vi "Export - Tx Packet.vi"(8 "error in (no error)":errorcluster, 11 "Device Item Ref in":T13 format="%.0x") -> (0 "error out":errorcluster, 3 "Tx Packet":T1 {"threadOptions"."pclDecimation" max=16 step=1; "threadOptions"."loopPeriod" max=16 step=1; "threadOptions"."targetPriority" min=-2 max=16 step=1; "threadOptions"."targetProcessor" min=-2 max=16 step=1; "Endianness" items=["big-endian"=0, "little-endian"=2]})   [LabVIEW 2019, in "UDP-Custom-Device System Explorer.lvlib"]
uses:
  UDP-Custom-Device System Explorer.lvlib
  <vilib>/NI VeriStand/Custom Device API/Custom Device Item Ref.ctl
  Types/XML - New/ImpExp - Tx Packet Data.ctl
  <vilib>/NI VeriStand/Custom Device API/Custom Device Item Info.ctl
  Shared/Types/Shared - Channel Data Type.ctl
  Shared/Types/Shared - Buffered.PacketInfo.ctl
  Shared/Types/Shared - Pointer Encoding.ctl
  Shared/Types/Shared - Receive Buffer Options.ctl
  Shared/Types/Shared - Transmit Buffer Options.ctl
  Shared/Types/Shared - Transmit Flag Options.ctl
  Shared/Types/Shared - Transmit Echo Options.ctl
  Types/Threading/Thread Configuration.ctl
  Types/Threading/Thread Sync Reference.ctl
  Shared/Types/Shared - Thread Management.ctl
  Property Accessors/Shared Packet Accessors.lvlib
  Property Accessors/Tx Packet Accessors.lvlib
  <vilib>/NI VeriStand/Custom Device API/Custom Device API.lvlib
  Shared/UDP-Custom-Device Shared.lvlib
  <vilib>/NI VeriStand/Custom Device Tools/Custom Device Utility Library/Custom Device Utility Library.lvlib
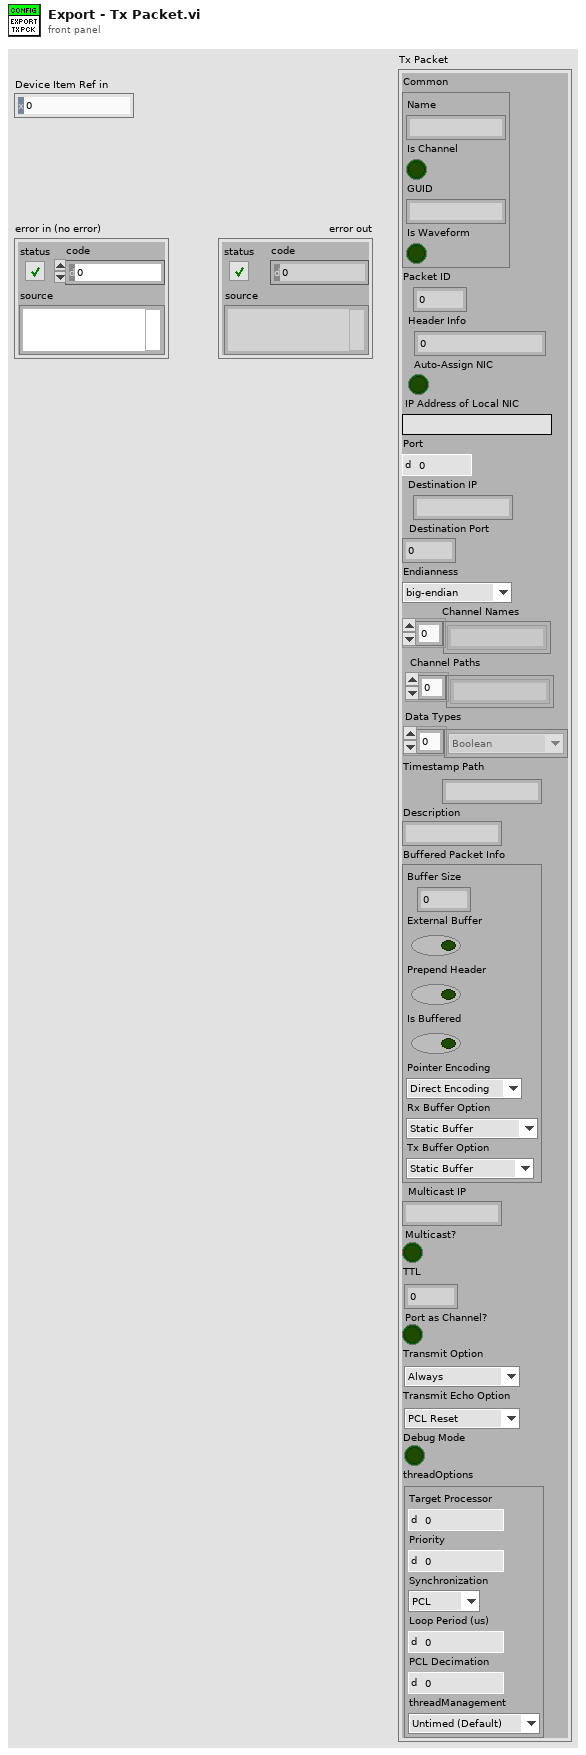
[diagram p1: front panel]
types:
  T1 = typedef "UDP-Custom-Device System Explorer.lvlib/ImpExp - Tx Packet Data.ctl" = cluster{"Common":T2, "Packet ID":i32, "Header Info":u32, "Auto-Assign NIC":bool, "IP Address of Local NIC":string, "Port":u16, "Destination IP":string, "Destination Port":u16, "Endianness":u16, "Channel Names":string[], "Channel Paths":string[], "Data Types":T3[], "Timestamp Path":string, "Description":string, "Buffered Packet Info":T4, "Multicast IP":string, "Multicast?":bool, "TTL":u16, "Port as Channel?":bool, "Transmit Option":T8, "Transmit Echo Option":T9, "Debug Mode":bool, "threadOptions":T10}
  T2 = typedef "Custom Device API.lvlib/Custom Device Item Info.ctl" = cluster{"Name":string, "Is Channel":bool, "GUID":string, "Is Waveform":bool}
  T3 = typedef "UDP-Custom-Device Shared.lvlib/Shared - Channel Data Type.ctl" = enum16{"Boolean", "Single", "Double", "I8", "I16", "I32", "I64", "U8", "U16", "U32", "U64"}
  T4 = typedef "UDP-Custom-Device Shared.lvlib/Shared - Buffered.PacketInfo.ctl" = cluster{"Buffer Size":i32, "External Buffer":bool, "Prepend Header":bool, "Is Buffered":bool, "Pointer Encoding":T5, "Rx Buffer Option":T6, "Tx Buffer Option":T7}
  T5 = typedef "UDP-Custom-Device Shared.lvlib/Shared - Pointer Encoding.ctl" = enum16{"Direct Encoding", "Conversion Encoding"}
  T6 = typedef "UDP-Custom-Device Shared.lvlib/Shared - Receive Buffer Options.ctl" = enum16{"Static Buffer", "Circular Buffer", "Circular Buffer + Size", "Internal Cache", "Internal Cache + Size", "Ping Pong", "Ping Pong + Size"}
  T7 = typedef "UDP-Custom-Device Shared.lvlib/Shared - Transmit Buffer Options.ctl" = enum16{"Static Buffer", "FIFO Buffer", "FIFO Buffer + Port"}
  T8 = typedef "UDP-Custom-Device Shared.lvlib/Shared - Transmit Flag Options.ctl" = enum16{"Always", "One-Shot", "Toggle"}
  T9 = typedef "UDP-Custom-Device Shared.lvlib/Shared - Transmit Echo Options.ctl" = enum16{"PCL Reset", "Counter", "Mirror"}
  T10 = typedef "UDP-Custom-Device System Explorer.lvlib/Thread Configuration.ctl" = cluster{"targetProcessor":i8, "targetPriority":i16, "Synchronization":T11, "loopPeriod":u32, "pclDecimation":u16, "threadManagement":T12}
  T11 = typedef "UDP-Custom-Device System Explorer.lvlib/Thread Sync Reference.ctl" = enum16{"PCL", "Async"}
  T12 = typedef "UDP-Custom-Device Shared.lvlib/Shared - Thread Management.ctl" = enum16{"Untimed (Default)", "Timed (High Priority)"}
  T13 = typedef "Custom Device API.lvlib/Custom Device Item Ref.ctl" = u64
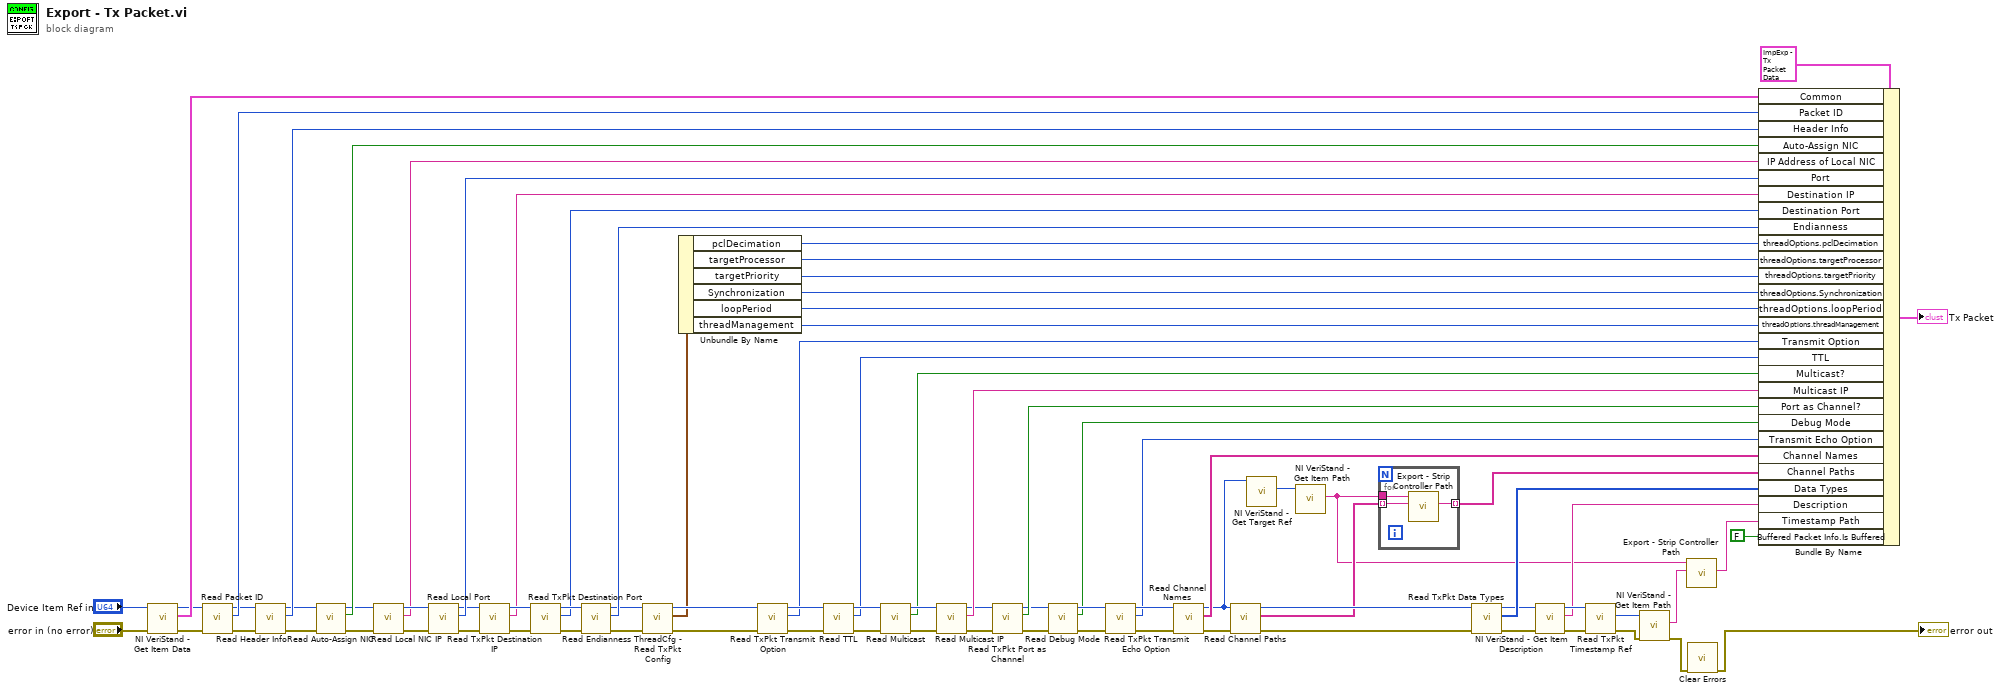
[diagram p0: block diagram]
diagram:
  n1 = call <vilib>:"NI VeriStand - Get Item Data.vi"("error in (no error)"="error in (no error)", "Item Ref in"="Device Item Ref in") -> ("error out"=w49:errorcluster, "Item Info"=w80:T2, "Item Ref out"=w79:T13)  [unwired: 6 in, 1 out]
  n2 = call "Read Packet ID.vi"("error in (no error)"=w49, "Node Ptr"=w79) -> ("error out"=w76:errorcluster, "Packet ID"=w78:i32, "Node Ptr out"=w77:T13)  [unwired: 7 in]
  n3 = call "Read Header Info.vi"("error in (no error)"=w76, "Node Ptr"=w77) -> ("error out"=w73:errorcluster, "Header Info"=w75:u32, "Node Ptr out"=w74:T13)  [unwired: 7 in]
  n4 = call "Read Auto-Assign NIC.vi"("error in (no error)"=w73, "Node Ptr"=w74) -> ("error out"=w68:errorcluster, "Auto-Assign NIC"=w72:bool, "Node Ptr out"=w71:T13)  [unwired: 7 in]
  n5 = call "Read Local NIC IP.vi"("error in (no error)"=w68, "Node Ptr"=w71) -> ("error out"=w69:errorcluster, "IP Address of Local NIC"=w67:string, "Node Ptr out"=w70:T13)  [unwired: 7 in]
  n6 = call "Read Local Port.vi"("error in (no error)"=w69, "Node Ptr"=w70) -> ("error out"=w64:errorcluster, "Port"=w66:u16, "Node Ptr out"=w65:T13)  [unwired: 7 in]
  n7 = call "Read TxPkt Destination IP.vi"("error in (no error)"=w64, "Node Ptr"=w65) -> ("error out"=w62:errorcluster, "Destination IP"=w59:string, "Node Ptr out"=w63:T13)  [unwired: 7 in]
  n8 = call "Read TxPkt Destination Port.vi"("error in (no error)"=w62, "Node Ptr"=w63) -> ("error out"=w60:errorcluster, "Destination Port"=w58:u16, "Node Ptr out"=w61:T13)  [unwired: 7 in]
  n9 = call "Read Endianness.vi"("error in (no error)"=w60, "Node Ptr"=w61) -> ("error out"=w8:errorcluster, "Endianness"=w57:u16, "Node Ptr out"=w9:T13)  [unwired: 7 in]
  n10 = call "ThreadCfg - Read TxPkt Config.vi"("error in (no error)"=w8, "Node Ptr In"=w9) -> ("error out"=w11:errorcluster, "threadOptions"=w7:T10, "Node Ptr Out"=w10:T13)  [unwired: 7 in]
  n11 = Unbundle By Name(w7) -> ("pclDecimation"=w6:u16, "targetProcessor"=w5:i8, "targetPriority"=w4:i16, "Synchronization"=w3:T11, "loopPeriod"=w2:u32, "threadManagement"=w1:T12)
  n12 = call "Read TxPkt Transmit Option.vi"("error in (no error)"=w11, "Node Ptr"=w10) -> ("error out"=w21:errorcluster, "Transmit Options"=w20:T8, "Node Ptr out"=w22:T13)  [unwired: 7 in]
  n13 = call "Read TTL.vi"("error in (no error)"=w21, "Node Ptr"=w22) -> ("error out"=w33:errorcluster, "TTL"=w29:u16, "Node Ptr out"=w32:T13)  [unwired: 7 in]
  n14 = call "Read Multicast.vi"("error in (no error)"=w33, "Node Ptr"=w32) -> ("error out"=w30:errorcluster, "Multicast"=w28:bool, "Node Ptr out"=w31:T13)  [unwired: 7 in]
  n15 = call "Read Multicast IP.vi"("error in (no error)"=w30, "Node Ptr"=w31) -> ("error out"=w24:errorcluster, "Multicast IP Address"=w27:string, "Node Ptr out"=w25:T13)  [unwired: 7 in]
  n16 = call "Read TxPkt Port as Channel.vi"("error in (no error)"=w24, "Node Ptr"=w25) -> ("error out"=w14:errorcluster, "Port as Channel"=w23:bool, "Node Ptr out"=w16:T13)  [unwired: 7 in]
  n17 = call "Read Debug Mode.vi"("error in (no error)"=w14, "Node Ptr"=w16) -> ("error out"=w13:errorcluster, "Debug Mode"=w12:bool, "Node Ptr out"=w15:T13)  [unwired: 7 in]
  n18 = call "Read TxPkt Transmit Echo Option.vi"("error in (no error)"=w13, "Node Ptr"=w15) -> ("error out"=w19:errorcluster, "Transmit Echo Options"=w17:T9, "Node Ptr out"=w18:T13)  [unwired: 7 in]
  n19 = call "Read Channel Names.vi"("error in (no error)"=w19, "Node Ptr"=w18) -> ("error out"=w56:errorcluster, "Channel Names"=w55:string[], "Node Ptr out"=w39:T13)  [unwired: 7 in]
  n20 = call "Read Channel Paths.vi"("error in (no error)"=w56, "Node Ptr"=w39) -> ("error out"=w53:errorcluster, "Channel Paths"=w38:string[], "Node Ptr out"=w54:T13)  [unwired: 7 in]
  n21 = call <vilib>:"NI VeriStand - Get Target Ref.vi"("Item Ref in"=w39) -> ("Target Ref"=w40:T13)  [unwired: 7 in, 3 out]
  n22 = call <vilib>:"NI VeriStand - Get Item Path.vi"("Item Ref in"=w40) -> ("Path"=w36:string)  [unwired: 7 in, 3 out]
  n23 = for {
    tunnel: w38 -> [w86] mode=indexing
    tunnel: w36 -> [w85]
    tunnel: [w84] -> w37 mode=indexing
    n24 = call "Export - Strip Controller Path.vi"("Channel Path"=w86, "Controller Path"=w85) -> ("Stripped Path"=w84:string)  [unwired: 8 in, 1 out]
  }
  n25 = call "Read TxPkt Data Types.vi"("error in (no error)"=w53, "Node Ptr"=w54) -> ("error out"=w43:errorcluster, "Data types"=w52:T3[], "Node Ptr out"=w45:T13)  [unwired: 7 in]
  n26 = call <vilib>:"NI VeriStand - Get Item Description.vi"("error in (no error)"=w43, "Item Ref in"=w45) -> ("error out"=w42:errorcluster, "Description"=w41:string, "Item Ref out"=w44:T13)  [unwired: 6 in, 1 out]
  n27 = call "Read TxPkt Timestamp Ref.vi"("error in (no error)"=w42, "Node Ptr"=w44) -> ("error out"=w50:errorcluster, "Timestamp Ref"=w51:T13)  [unwired: 7 in, 1 out]
  n28 = call <vilib>:"NI VeriStand - Get Item Path.vi"("error in (no error)"=w50, "Item Ref in"=w51) -> ("error out"=w48:errorcluster, "Path"=w35:string)  [unwired: 6 in, 2 out]
  n29 = call "Export - Strip Controller Path.vi"("Channel Path"=w35, "Controller Path"=w36) -> ("Stripped Path"=w34:string)  [unwired: 8 in, 1 out]
  n30 = call <vilib>:"Clear Errors.vi"("error in (no error)"=w48) -> ("error out"=→"error out":errorcluster)  [unwired: 5 in, 1 out]
  n31 = Bundle By Name(cluster=T1 {"Common"={"Name"="", "Is Channel"=FALSE, "GUID"="", "Is Waveform"=FALSE}, "Packet ID"=0, "Header Info"=0, "Auto-Assign NIC"=FALSE, "IP Address of Local NIC"="", "Port"=0, "Destination IP"="", "Destination Port"=0, "Endianness"=0, "Channel Names"=[], "Channel Paths"=[], "Data Types"=[], "Timestamp Path"="", "Description"="", "Buffered Packet Info"={"Buffer Size"=0, "External Buffer"=FALSE, "Prepend Header"=FALSE, "Is Buffered"=FALSE, "Pointer Encoding"=enum."Direct Encoding", "Rx Buffer Option"=enum."Static Buffer", "Tx Buffer Option"=enum."Static Buffer"}, "Multicast IP"="", "Multicast?"=FALSE, "TTL"=0, "Port as Channel?"=FALSE, "Transmit Option"=enum."Always", "Transmit Echo Option"=enum."PCL Reset", "Debug Mode"=FALSE, "threadOptions"={"targetProcessor"=0, "targetPriority"=0, "Synchronization"=enum."PCL", "loopPeriod"=0, "pclDecimation"=0, "threadManagement"=enum."Untimed (Default)"}} ("Tx Packet"), "Common"=w80, "Packet ID"=w78, "Header Info"=w75, "Auto-Assign NIC"=w72, "IP Address of Local NIC"=w67, "Port"=w66, "Destination IP"=w59, "Destination Port"=w58, "Endianness"=w57, "threadOptions.pclDecimation"=w6, "threadOptions.targetProcessor"=w5, "threadOptions.targetPriority"=w4, "threadOptions.Synchronization"=w3, "threadOptions.loopPeriod"=w2, "threadOptions.threadManagement"=w1, "Transmit Option"=w20, "TTL"=w29, "Multicast?"=w28, "Multicast IP"=w27, "Port as Channel?"=w23, "Debug Mode"=w12, "Transmit Echo Option"=w17, "Channel Names"=w55, "Channel Paths"=w37, "Data Types"=w52, "Description"=w41, "Timestamp Path"=w34, "Buffered Packet Info.Is Buffered"=FALSE) -> (→"Tx Packet":T1)
